vi "Get File Extension.vi"(8 "Error In":errorcluster, 11 "File Path Control":path) -> (0 "Error Out":errorcluster, 2 "Extension":string, 3 "Duplicate Path":path)   [LabVIEW 2014, in "LMH-Toolbox.lvlib"]
doc: "This VI returns the file extension of the specified file."
uses:
  <vilib>/MakerHub/Toolbox/LMH-Toolbox.lvlib
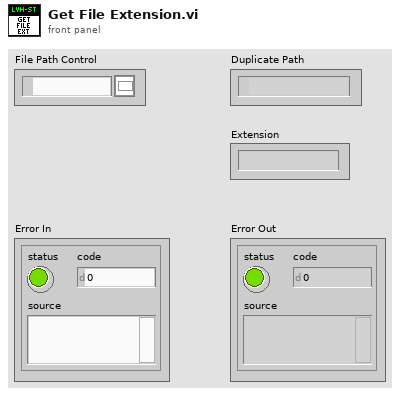
[diagram p1: front panel]
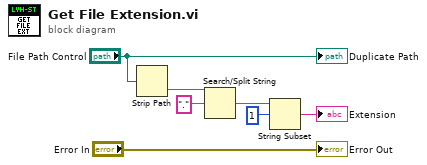
[diagram p0: block diagram]
diagram:
  n1 = Strip Path(path="File Path Control") -> (name=w1:string)  [unwired: 1 out]
  n2 = Search/Split String(string=w1, search string/char (-)=".") -> (match + rest of string=w6:string)  [unwired: 1 in, 2 out]
  n3 = String Subset(string=w6, offset (0)=1) -> (substring=→"Extension":string)  [unwired: 1 in]
  "Duplicate Path" <- "File Path Control"
  "Error Out" <- "Error In"
